vi "Day 3.1 - Calculate rates.vi"(11 "input":string[](array[string])) -> (3 "output":u32)   [LabVIEW 2021]
panel:
  out "Epsilon":u32
  out "Gamma":u32
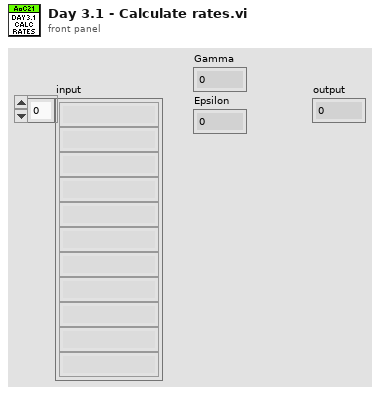
[diagram p1: front panel]
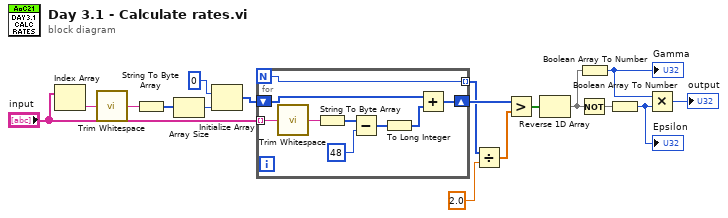
[diagram p0: block diagram]
diagram:
  n1 = Index Array(array="input") -> (element=w15:string)  [unwired: 1 in]
  n2 = call <vilib>:"Trim Whitespace.vi"("string"=w15) -> ("trimmed string"=w16:string)  [unwired: 1 in]
  n3 = String To Byte Array(string=w16) -> (unsigned byte array=w14:u8[])
  n4 = Array Size(array=w14) -> (size(s)=w13:i32)
  n5 = Initialize Array(0, w13) -> (w11:i32[])
  n6 = for {
    N -> [w18]
    tunnel: "input" -> [w26] mode=indexing
    shift-right: [w23] -> w10
    shift-left: w11 -> [w24]
    tunnel: [w18] -> w1 mode=indexing
    n7 = call <vilib>:"Trim Whitespace.vi"("string"=w26) -> ("trimmed string"=w25:string)  [unwired: 1 in]
    n8 = String To Byte Array(string=w25) -> (unsigned byte array=w22:u8[])
    n9 = Subtract(x=w22, y=u8 48) -> (x-y=w20:u8[])
    n10 = To Long Integer(number=w20) -> (32bit integer=w21:i32[])
    n11 = Add(x=w24, y=w21) -> (x+y=w23:i32[])
  }
  n12 = Divide(x=w1, y=2.0) -> (x/y=w2:dbl[])
  n13 = Greater?(x=w10, y=w2) -> (0:w8:bool[])
  n14 = Reverse 1D Array(array=w8) -> (reversed array=w5:bool[])
  n15 = Not(x=w5) -> (.not. x?=w4:bool[])
  n16 = Boolean Array To Number(Boolean array=w5) -> (number=w7:u32)
  "Gamma" <- w7
  n17 = Boolean Array To Number(Boolean array=w4) -> (number=w3:u32)
  "Epsilon" <- w3
  n18 = Multiply(x=w7, y=w3) -> (x*y=→"output":u32)
